vi "Wait Sampling Done.vi"(4 "stop notifier ref (none)":refnum<notifier>, 6 "stop ref (none)":refnum<vi>, 7 "semaphore":T1, 8 "error in":errorcluster, 10 "timeout [s] (5s)":dbl=5.0, 11 "VISA resource in":refnum<visa-resource-name>) -> (0 "error out":errorcluster, 3 "VISA resource out":refnum<visa-resource-name>)   [LabVIEW 2018, in "3458A Virtual Digitizer.lvlib" / "3458A Digitizing Low Levels.lvlib"]
doc: "This VI checks status of the DMM while it is digitizing. It waits until NRDGS defined number of samples is digitized, then it returns. The waiting has timeout option. When timeout is reached it will generate error. It can be also terminated by reference to boolean variable, i.e. if the variable is True. Another way to terminate it is boolean notifier. If the notification is detected and the message content is True it terminates the wait loop.\nIf the waiting was aborted by timeout or stop or error it will return True at 'was aborted?' output.\n\nNote: Reentrant VI so it can be executed in parallel for multiple 3458A sessions."
uses:
  3458A Digitizing Low Levels.lvlib
  <vilib>/Utility/error.llb/Error Cluster From Error Code.vi
  <vilib>/ErrorRing/Error Ring.xnode
  3458A Basic Driver/3458A Basic Driver.lvlib
panel:
  out "was aborted?":bool
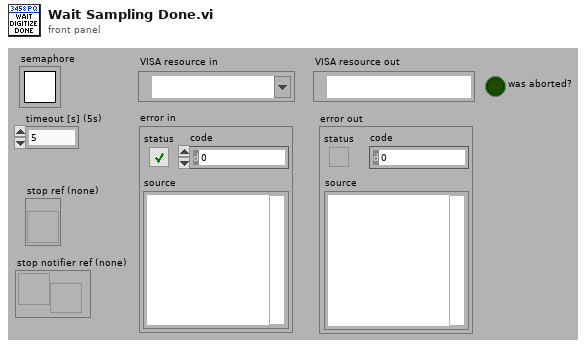
[diagram p1: front panel]
types:
  T1 = typedef "Semaphore RefNum" = refnum<k1>
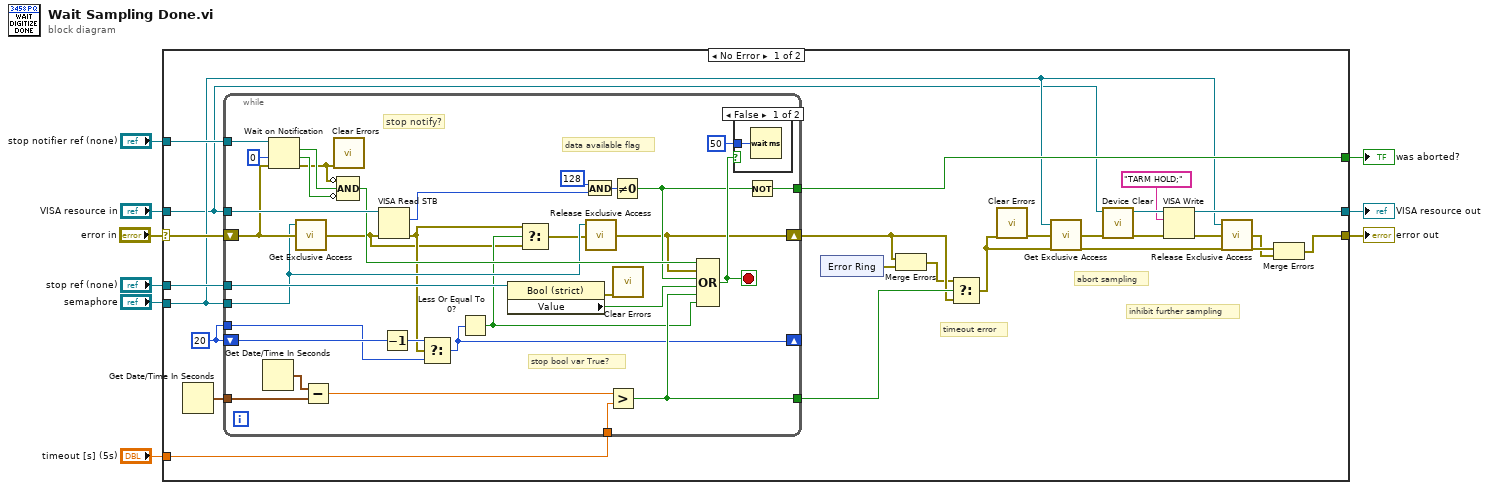
[diagram p0: block diagram]
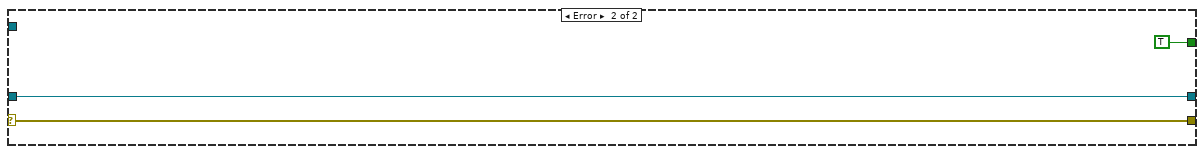
[diagram p3: hidden frame]
diagram:
  n1 = case shown="No Error" "error in" {
    selector: "error in" -> [w31 w74]
    tunnel: [w18 w74] -> w7
    tunnel: "VISA resource in" -> [w11 w73]
    tunnel: [w17 w73] -> w6
    tunnel: "stop ref (none)" -> [w32 _]
    tunnel: "timeout [s] (5s)" -> [w29 _]
    tunnel: "stop notifier ref (none)" -> [w24 _]
    tunnel: [w19 TRUE] -> w2
    tunnel: "semaphore" -> [w12 _]
    frame No Error {
      w10 = 20
      # "inhibit further sampling"
      # "abort sampling"
      # "timeout error"
      n2 = Get Date/Time In Seconds() -> (seconds since 1Jan1904=w30:timestamp)
      n3 = while {
        shift-right: [w47] -> w26
        shift-left: w31 -> [w48]
        tunnel: w32 -> [w66]
        tunnel: w30 -> [w59]
        tunnel: w29 -> [w60]
        tunnel: [w57] -> w28
        tunnel: w24 -> [w56]
        tunnel: [w50] -> w19
        tunnel: w12 -> [w46]
        tunnel: w11 -> [w70]
        shift-right: [w42] -> _
        shift-left: w10 -> [w45]
        tunnel: w10 -> [w43]
        stop <- w62 stop-if-true
        # "stop bool var True?"
        # "stop notify?"
        # "data available flag"
        n4 = Get Date/Time In Seconds() -> (seconds since 1Jan1904=w58:timestamp)
        n5 = Wait on Notification(notifier=w56, timeout in ms (-1)=0, error in (no error)=w48) -> (notification=w54:bool, timed out?=w55:bool, error out=w53:errorcluster)  [unwired: 1 in, 1 out]
        n6 = call "Get Exclusive Access.vi"("semaphore"=w46, "error in (no error)"=w48) -> ("error out"=w38:errorcluster)  [unwired: 7 in]
        n7 = Subtract(x=w58, y=w59) -> (x-y=w61:dbl)
        n8 = call <vilib>:"Clear Errors.vi"("error in (no error)"=w53) -> ()  [unwired: 5 in, 2 out]
        n9 = Compound Arithmetic op=AND(invert w53, w54, invert w55) -> (w52:bool)
        n10 = VISA Read STB(8:w38, 11:w70) -> (0:w40:errorcluster, 2:w69:u16)  [unwired: 1 out]
        n11 = Decrement(x=w45) -> (x-1=w44:i32)
        n12 = Select(t=w44, s=w40, f=w43) -> (s? t:f=w42:i32)
        n13 = Less Or Equal To 0?(x=w42) -> (x <= 0?=w41:bool)
        n14 = property class="Bool (strict)"(reference=w66) -> (error out=w64:errorcluster, "Value"=w65:bool)  [unwired: 1 in, 1 out]
        n15 = Select(t=w40, s=w41, f=w38) -> (s? t:f=w39:errorcluster)
        n16 = And(x=u16 128, y=w69) -> (x .and. y?=w67:u16)
        n17 = call "Release Exclusive Access.vi"("semaphore"=w46, "error in (no error)"=w39) -> ("error out"=w47:errorcluster)  [unwired: 7 in]
        n18 = Greater?(x=w61, y=w60) -> (0:w57:bool)
        n19 = Not Equal To 0?(x=w67) -> (x != 0?=w51:bool)
        n20 = call <vilib>:"Clear Errors.vi"("error in (no error)"=w64) -> ()  [unwired: 5 in, 2 out]
        n21 = Compound Arithmetic op=OR(w52, w47, w51, w65, w57, w41) -> (w62:bool)
        n22 = case shown="False" w62 {
          tunnel: u32 50 ("milliseconds to wait") -> [w71 _]
          frame False {
            n23 = Wait (ms)(milliseconds to wait=w71) -> ()  [unwired: 1 out]
          }
          frame True {
          }
        }
        n24 = Not(x=w51) -> (.not. x?=w50:bool)
      }
      n25 = xnode "Error Ring"() -> ("error out"=w27:errorcluster)
      n26 = Merge Errors(w26, w27) -> (w25:errorcluster)
      n27 = Select(t=w25, s=w28, f=w26) -> (s? t:f=w20:errorcluster)
      n28 = call <vilib>:"Clear Errors.vi"("error in (no error)"=w20) -> ("error out"=w16:errorcluster)  [unwired: 5 in, 1 out]
      n29 = call "Get Exclusive Access.vi"("semaphore"=w12, "error in (no error)"=w16) -> ("error out"=w15:errorcluster)  [unwired: 7 in]
      n30 = call "Device Clear.vi"("error in(no error)"=w15, "VISA Resource Name"=w11) -> ("error out"=w22:errorcluster, "VISA resource name out"=w23:refnum<visa-resource-name>)  [unwired: 8 in]
      n31 = VISA Write(VISA resource name=w23, write buffer="TARM HOLD;", error in (no error)=w22) -> (VISA resource name out=w17:refnum<visa-resource-name>, error out=w14:errorcluster)  [unwired: 1 out]
      n32 = call "Release Exclusive Access.vi"("semaphore"=w12, "error in (no error)"=w14) -> ("error out"=w13:errorcluster)  [unwired: 7 in]
      n33 = Merge Errors(w20, w13) -> (w18:errorcluster)
    }
    frame Error {
    }
  }
  "VISA resource out" <- w6
  "error out" <- w7
  "was aborted?" <- w2
